vi "CAD@SetRobotPosByPoint__Parameter.vi"(1 "ParamterIn":string) -> (0 "ParamterOut":string)   [LabVIEW 2019]
panel:
  in  "RobotName":string(combo)
  in  "Confirm":bool
  # "CAD@SetRobotPosByPoint $Robot"
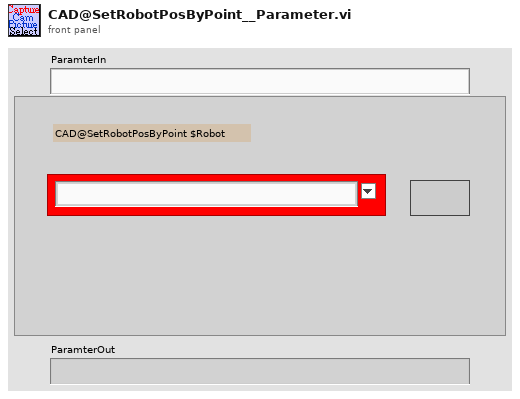
[diagram p1: front panel]
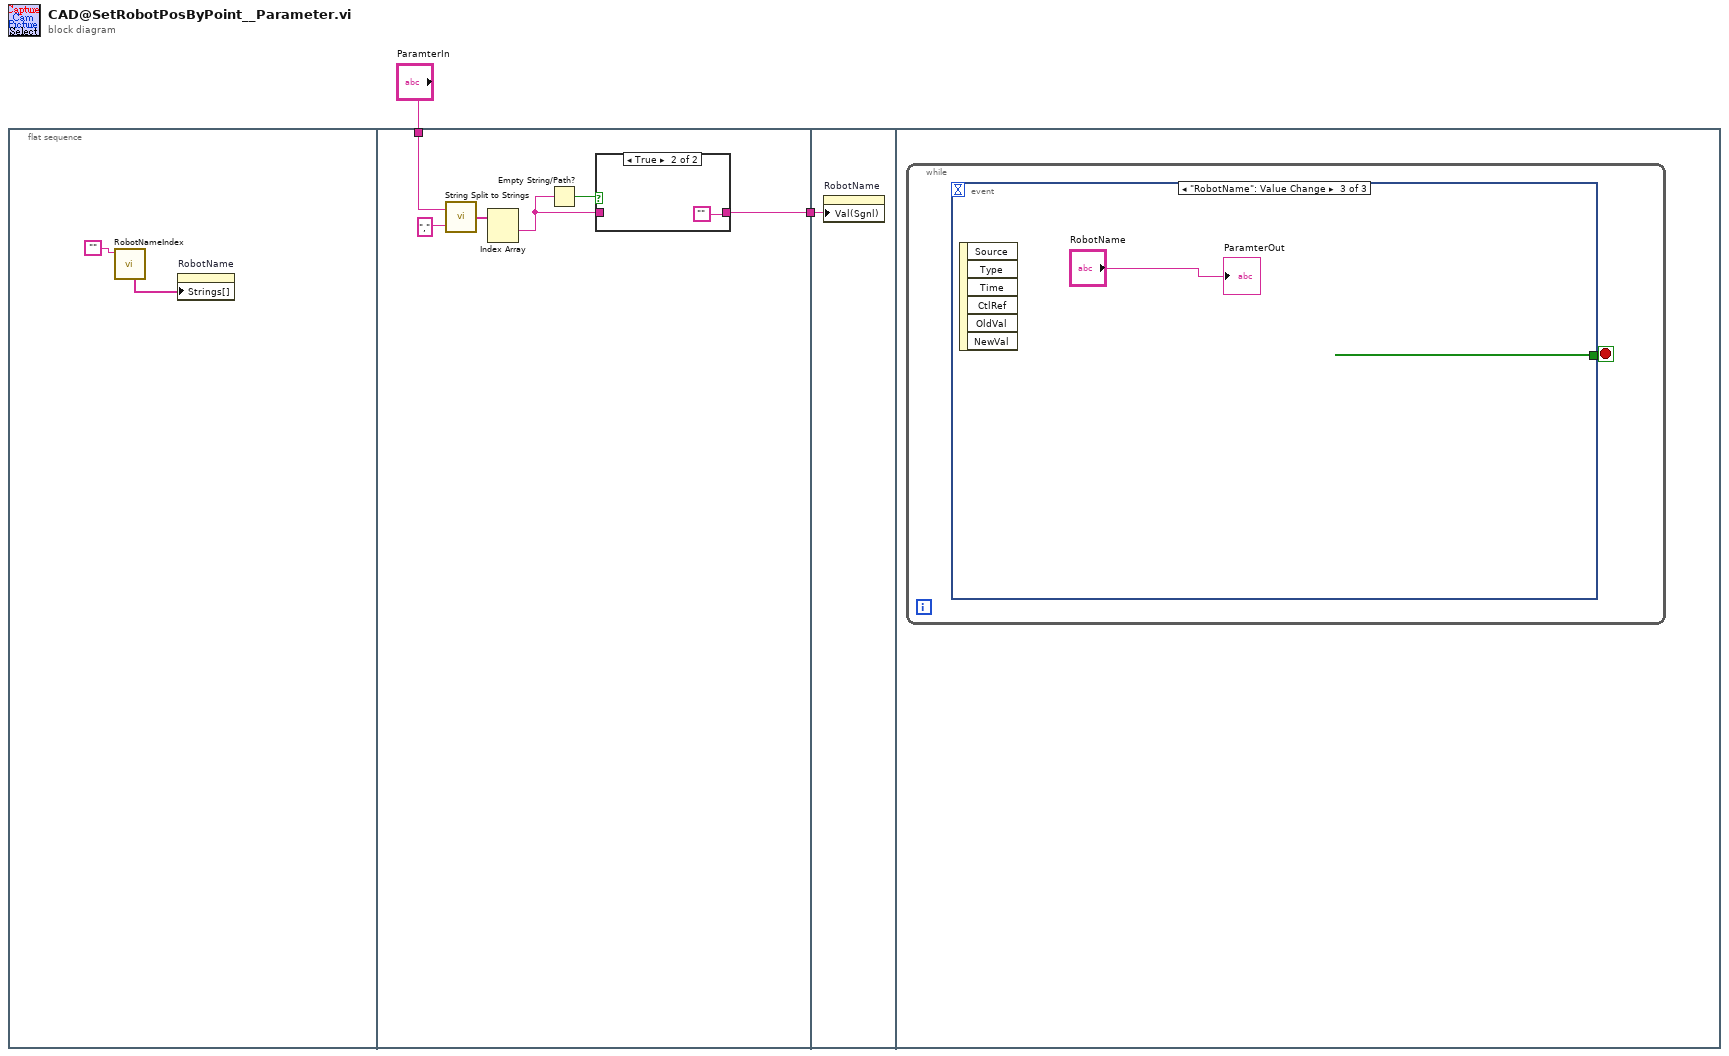
[diagram p0: block diagram]
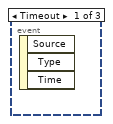
[diagram p3: hidden frame]
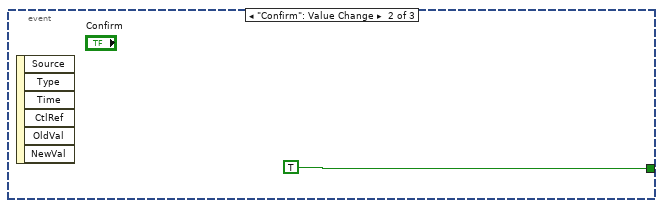
[diagram p4: hidden frame]
diagram:
  n1 = flat-sequence {
    tunnel: "ParamterIn" -> [w8]
    tunnel: [w5] -> w1
    tunnel: w1 -> [w13]
    frame #0 {
      n2 = call "RobotNameIndex.vi"("RobotName"="") -> ("RobotNameList"=w3:string[])  [unwired: 8 in, 2 out]
      n3 = property on="RobotName" class="CmbBox"("Strings[]"=w3) -> ()  [unwired: 2 in, 2 out]
    }
    frame #1 {
      n4 = call "String Split to Strings.vi"("search string/char (-)"=",", "String"=w8) -> ("Array"=w10:string[])
      n5 = Index Array(array=w10) -> (element #1=w6:string)  [unwired: 2 in, 1 out]
      n6 = Empty String/Path?(string/path=w6) -> (empty?=w7:bool)
      n7 = case shown="True" w7 {
        tunnel: w6 -> [w11 _]
        tunnel: [w11 ""] -> w5
        frame False {
        }
        frame True {
        }
      }
    }
    frame #2 {
      n8 = property on="RobotName" class="CmbBox"("Val(Sgnl)"=w13) -> ()  [unwired: 2 in, 2 out]
    }
    frame #3 {
      n9 = while {
        stop <- w14 stop-if-true
        n10 = event shown="[2] \"RobotName\": Value Change" {
          selector: _ -> [_ _ _]
          dyn-events: _ -> [_ _ _]
          timeout: _ -> [_ _ _]
          tunnel: [_ TRUE _] -> w14
          event Timeout {
            n11 = event-data() -> ()  [unwired: 1 in, 3 out]
          }
          event "Confirm": Value Change {
            n12 = event-data() -> ()  [unwired: 1 in, 6 out]
          }
          event "RobotName": Value Change {
            n13 = event-data() -> ()  [unwired: 1 in, 6 out]
            "ParamterOut" <- "RobotName"
          }
        }
      }
    }
  }
